vi "RasgeleSayılarıDiziyeKaydedenProgram.vi"() -> ()   [LabVIEW 2014]
panel:
  out "Array":dbl[](array[numeric])
  # "0 ile 6 arasında rasgele 5 sayı üretip bu sayıları bir \ndiziye kaydeden program."
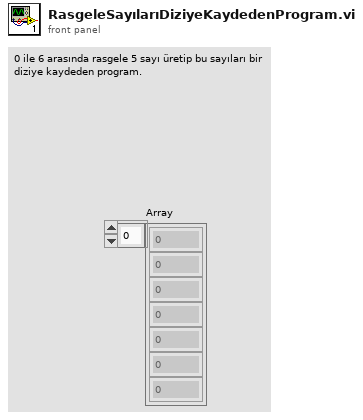
[diagram p1: front panel]
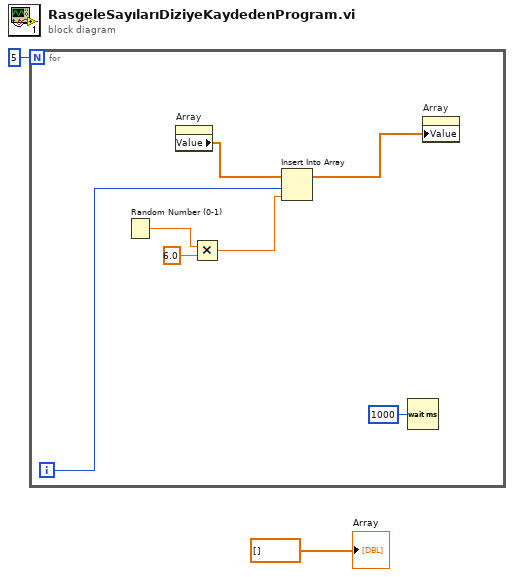
[diagram p0: block diagram]
diagram:
  n1 = for {
    N: 5 -> [_]
    i -> [w6]
    n2 = Random Number (0-1)() -> (number: 0 to 1=w9:dbl)
    n3 = property on="Array" class="Arr (strict)"() -> ("Value"=w5:dbl[])  [unwired: 2 in, 2 out]
    n4 = Multiply(x=w9, y=6.0) -> (x*y=w7:dbl)
    n5 = Insert Into Array(array=w5, index=w6, new element=w7) -> (w3:dbl[])
    n6 = Wait (ms)(milliseconds to wait=u32 1000) -> ()  [unwired: 1 out]
    n7 = property on="Array" class="Arr (strict)"("Value"=w3) -> ()  [unwired: 2 in, 2 out]
  }
  "Array" <- dbl[] [] ("Array")
